vi "RT Main.vi"   [LabVIEW 2014]
uses:
  <vilib>/nisyscfg/nisyscfg.lvlib
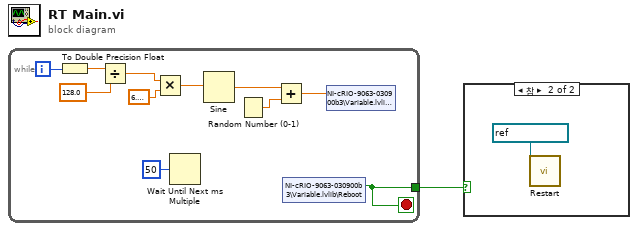
[diagram p0: block diagram]
diagram:
  n1 = while {
    tunnel: [w3] -> w1
    i -> [w12]
    stop <- w3 stop-if-true
    n2 = To Double Precision Float(number=w12) -> (double precision float=w11:dbl)
    n3 = Divide(x=w11, y=128.0) -> (x/y=w8:dbl)
    n4 = Multiply(x=w8, y=6.283185307179586) -> (x*y=w7:dbl)
    n5 = Wait Until Next ms Multiple(millisecond multiple=u32 50 ("ms 배수")) -> ()  [unwired: 1 out]
    n6 = Sine(x=w7) -> (sin(x)=w6:dbl)
    n7 = Random Number (0-1)() -> (number: 0 to 1=w5:dbl)
    n8 = Add(x=w6, y=w5) -> (x+y=w4:dbl)
    n9 = shared-variable "NI-cRIO-9063-030900b3\\Variable.lvlib\\Reboot"() -> (w3:bool)  [unwired: 1 in, 1 out]
    n10 = shared-variable "NI-cRIO-9063-030900b3\\Variable.lvlib\\Data"(w4) -> ()  [unwired: 1 in, 1 out]
  }
  n11 = case shown="참" w1 {
    frame False {
    }
    frame True {
      n12 = call <vilib>:"Restart.vi"("Session in"=refnum<k21> "localhost") -> ()  [unwired: 8 in, 3 out]
    }
  }
